vi "add_values.vi"(8 "F values array":dbl[][](array[numeric]), 9 "Values":dbl[](array[numeric]), 10 "Frekans":dbl, 11 "LstBox Refnum":refnum<vi>) -> (3 "Output F values array":dbl[][](array[numeric]))   [LabVIEW 2014]
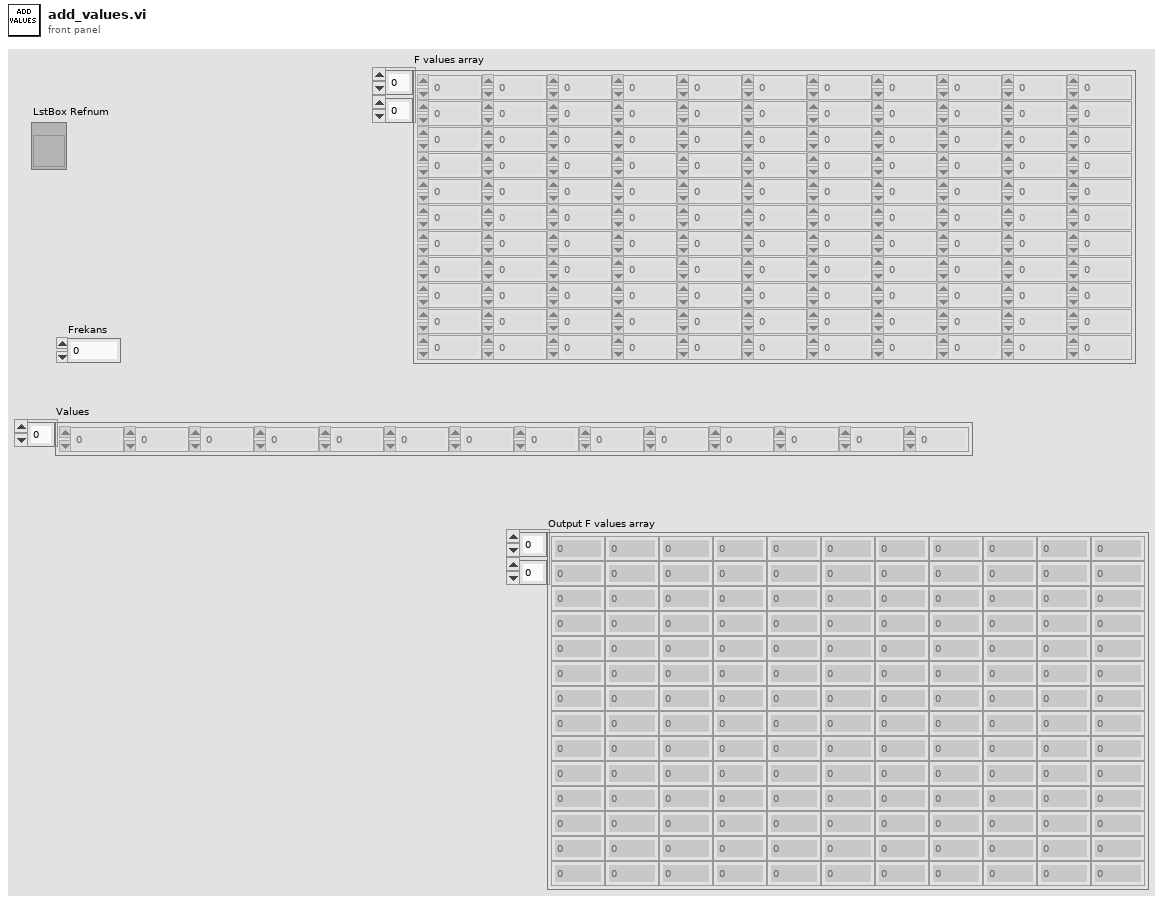
[diagram p1: front panel]
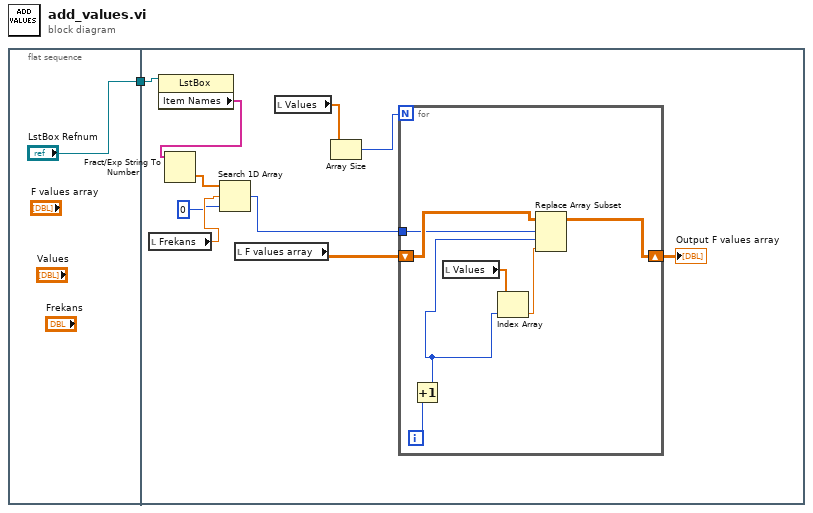
[diagram p0: block diagram]
diagram:
  n1 = flat-sequence {
    tunnel: ["LstBox Refnum"] -> w1
    tunnel: w1 -> [w4]
    frame #0 {
    }
    frame #1 {
      n2 = local read "Frekans"() -> (w10:dbl)
      n3 = property class="LstBox"(reference=w4) -> ("Item Names"=w5:string[])  [unwired: 1 in, 2 out]
      n4 = Fract/Exp String To Number(string=w5) -> (number=w11:dbl[])  [unwired: 3 in, 1 out]
      n5 = Search 1D Array(1D array=w11, element=w10, start index (0)=0) -> (index of element=w8:i32)
      n6 = local read "F values array"() -> (w12:dbl[][])
      n7 = local read "Values"() -> (w7:dbl[])
      n8 = Array Size(array=w7) -> (size(s)=w6:i32)
      n9 = for {
        N: w6 -> [_]
        shift-right: [w15] -> w3
        shift-left: w12 -> [w19]
        tunnel: w8 -> [w18]
        i -> [w14]
        n10 = Increment(x=w14) -> (x+1=w13:i32)
        n11 = local read "Values"() -> (w17:dbl[])
        n12 = Index Array(array=w17, index=w13) -> (element=w16:dbl)
        n13 = Replace Array Subset(array=w19, new element=w16, index (row)=w18, index (col)=w13) -> (w15:dbl[][])
      }
      "Output F values array" <- w3
    }
  }
